vi "ClusterWithActiveXRef.vi"(10 "Cluster":T1={"Numeric"=0.0, "String"="", "Cluster"={"Numeric"=0.0, "Cluster"={"Boolean"=FALSE, "Ring"=11}}} {"Cluster"."Cluster"."Ring" items=["aaaa"=11, "bbbb"=22, "cccc"=33]}, 11 "SequenceContext":refnum<k7>) -> (0 "error out":errorcluster, 3 "Has Expected Values":bool)   [LabVIEW 2012]
uses:
  <vilib>/addons/TestStand/_TSUtility.llb/TestStand - Get Property Value (Number).vi
  <vilib>/addons/TestStand/_TSUtility.llb/TestStand - Get Property Value (String).vi
  <vilib>/addons/TestStand/_TSUtility.llb/TestStand - Get Property Value (Boolean).vi
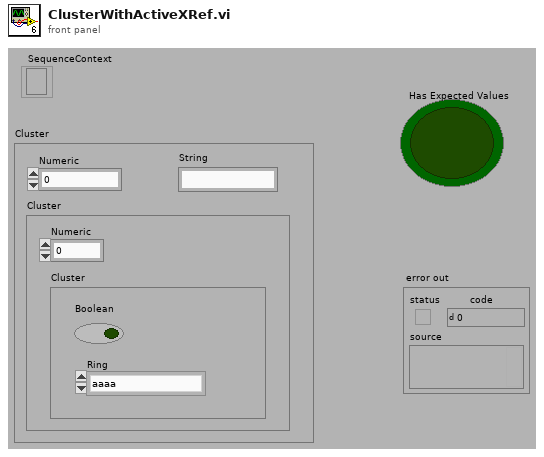
[diagram p1: front panel]
types:
  T1 = cluster{"Numeric":dbl, "String":string, "Cluster":cluster{"Numeric":dbl, "Cluster":cluster{"Boolean":bool, "Ring":u16}}}
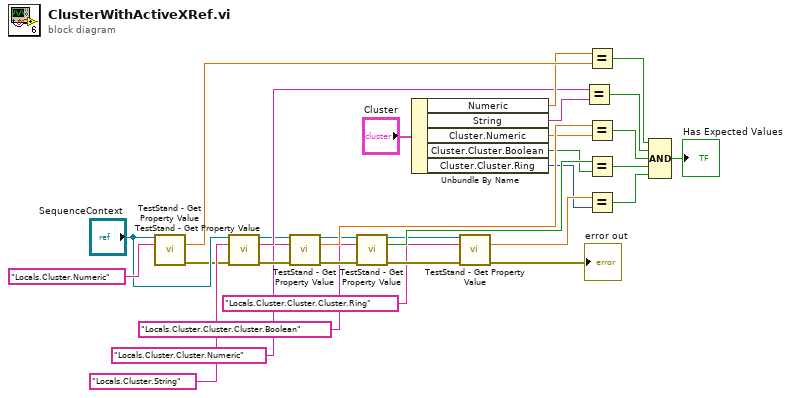
[diagram p0: block diagram]
diagram:
  n1 = call-poly <vilib>:"TestStand - Get Property Value.vi"("Sequence Context In"="SequenceContext", "Lookup String"="Locals.Cluster.Numeric") -> ("Value"=w28:dbl, "error out"=w19:errorcluster)  [unwired: 11 in, 1 out]
  n2 = call-poly <vilib>:"TestStand - Get Property Value.vi"("Sequence Context In"="SequenceContext", "Lookup String"="Locals.Cluster.String", "error in (no error)"=w19) -> ("Sequence Context Out"=w1:refnum<k7>, "Value"=w24:string, "error out"=w18:errorcluster)  [unwired: 10 in]
  n3 = call-poly <vilib>:"TestStand - Get Property Value.vi"("Sequence Context In"=w1, "Lookup String"="Locals.Cluster.Cluster.Numeric", "error in (no error)"=w18) -> ("Sequence Context Out"=w2:refnum<k7>, "Value"=w15:dbl, "error out"=w20:errorcluster)  [unwired: 10 in]
  n4 = call-poly <vilib>:"TestStand - Get Property Value.vi"("Sequence Context In"=w2, "Lookup String"="Locals.Cluster.Cluster.Cluster.Boolean", "error in (no error)"=w20) -> ("Sequence Context Out"=w3:refnum<k7>, "Value"=w12:bool, "error out"=w17:errorcluster)  [unwired: 10 in]
  n5 = Unbundle By Name("Cluster") -> ("Numeric"=w27:dbl, "String"=w23:string, "Cluster.Numeric"=w14:dbl, "Cluster.Cluster.Boolean"=w11:bool, "Cluster.Cluster.Ring"=w6:u16)
  n6 = call-poly <vilib>:"TestStand - Get Property Value.vi"("Sequence Context In"=w3, "Lookup String"="Locals.Cluster.Cluster.Cluster.Ring", "error in (no error)"=w17) -> ("Value"=w7:dbl, "error out"=→"error out":errorcluster)  [unwired: 10 in, 1 out]
  n7 = Equal?(x=w24, y=w23) -> (x = y?=w22:bool)
  n8 = Equal?(x=w27, y=w28) -> (x = y?=w26:bool)
  n9 = Equal?(x=w15, y=w14) -> (x = y?=w10:bool)
  n10 = Equal?(x=w12, y=w11) -> (x = y?=w9:bool)
  n11 = Equal?(x=w7, y=w6) -> (x = y?=w5:bool)
  n12 = Compound Arithmetic op=AND(w26, w22, w10, w9, w5) -> (→"Has Expected Values":bool)
